vi "Colorcycle2000.vi"   [LabVIEW 2013]
uses:
  <vilib>/Heliosphere Research LLC/Advanced Plotting Toolkit/api_plotting/LineProperties.ctl
  <vilib>/Heliosphere Research LLC/Advanced Plotting Toolkit/properties/Line.ctl
  <vilib>/Heliosphere Research LLC/Advanced Plotting Toolkit/properties/Line_Style.ctl
  <vilib>/Heliosphere Research LLC/Advanced Plotting Toolkit/typedefs/PlotColor.ctl
  <vilib>/Heliosphere Research LLC/Advanced Plotting Toolkit/properties/Marker.ctl
  <vilib>/Heliosphere Research LLC/Advanced Plotting Toolkit/properties/Marker_Style.ctl
  <vilib>/Heliosphere Research LLC/Advanced Plotting Toolkit/properties/Display.ctl
  <vilib>/Heliosphere Research LLC/Advanced Plotting Toolkit/Advanced Plotting Toolkit.lvlib
types:
  T1 = typedef "Advanced Plotting Toolkit.lvlib/LineProperties.ctl" = cluster{"Line":T2, "Marker":T5, "Display":T7}
  T2 = typedef "Advanced Plotting Toolkit.lvlib/Line.ctl" = cluster{"Style":T3, "Color":T4, "Width":sgl}
  T3 = typedef "Advanced Plotting Toolkit.lvlib/Line_Style.ctl" = enum16{"Automatic", "Solid", "Dashed", "Dotted", "Dash-dot", "Invisible"}
  T4 = typedef "Advanced Plotting Toolkit.lvlib/PlotColor.ctl" = u32
  T5 = typedef "Advanced Plotting Toolkit.lvlib/Marker.ctl" = cluster{"Style":T6, "Color":T4, "Size":dbl}
  T6 = typedef "Advanced Plotting Toolkit.lvlib/Marker_Style.ctl" = enum16{"Automatic", "Circle", "Square", "Triangle", "Diamond", "Star", "Invisible"}
  T7 = typedef "Advanced Plotting Toolkit.lvlib/Display.ctl" = cluster{"Alpha":dbl, "Z Order":dbl}
  T8 = typedef "Advanced Plotting Toolkit.lvlib/PlotID.ctl" = i32
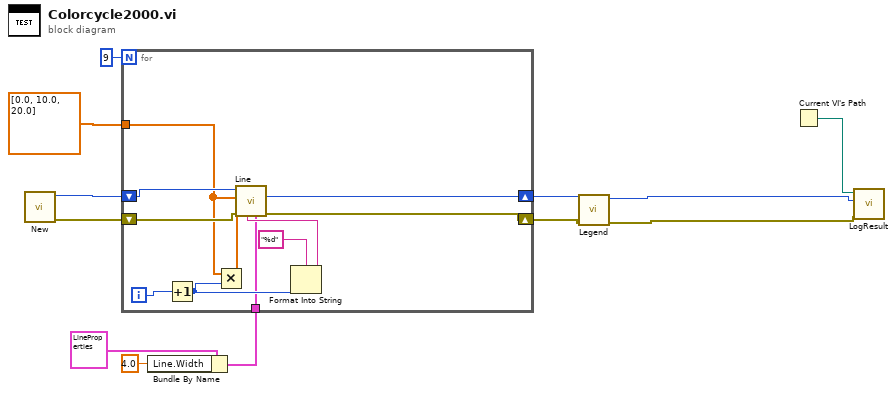
[diagram p0: block diagram]
diagram:
  n1 = call <vilib>:"New.vi"() -> ("error out"=w9:errorcluster, "Plot ID"=w11:T8)  [unwired: 10 in]
  n2 = Bundle By Name(cluster=T1 {"Line"={"Style"=enum."Automatic", "Color"=2147483647, "Width"=nan}, "Marker"={"Style"=enum."Automatic", "Color"=2147483647, "Size"=nan}, "Display"={"Alpha"=nan, "Z Order"=nan}} ("Line Plot Properties"), "Line.Width"=sgl 4.0) -> (w2:T1)
  n3 = for {
    N: 9 -> [_]
    shift-right: [w20] -> w8
    shift-left: w11 -> [w23]
    tunnel: dbl[] [0.0, 10.0, 20.0] -> [w18]
    shift-right: [w21] -> w6
    shift-left: w9 -> [w22]
    tunnel: w2 -> [w13]
    i -> [w19]
    n4 = Increment(x=w19) -> (x+1=w15:i32)
    n5 = Multiply(x=w18, y=w15) -> (x*y=w17:dbl[])
    n6 = Format Into String(format string="%d", w15) -> (resulting string=w14:string)  [unwired: 2 in, 1 out]
    n7 = call <vilib>:"Line.vi"("Properties"=w13, "Legend Title"=w14, "error in (no error)"=w22, "Y Data"=w17, "X Data"=w18, "Plot ID"=w23) -> ("error out"=w21:errorcluster, "Plot ID out"=w20:T8)  [unwired: 4 in]
  }
  n8 = call <vilib>:"Legend.vi"("error in (no error)"=w6, "Plot ID"=w8) -> ("error out"=w5:errorcluster, "Plot ID Out"=w7:T8)  [unwired: 8 in]
  n9 = Current VI's Path() -> (path=w12:path)
  n10 = call "LogResult.vi"("Test Result"=w5, "Test Artifact"=w7, "VI Path"=w12) -> ()  [unwired: 9 in]
